vi "Display Results.vi"(8 "error in (no error)":errorcluster, 11 "Freq Sweet Result in":refnum<class "Freq Sweep Result.lvclass">) -> (0 "error out":errorcluster, 3 "Freq Sweet Result out":refnum<class "Freq Sweep Result.lvclass">)   [LabVIEW 2015, in "Frequency Measurement.lvlib" / "Freq Sweep Result.lvclass"]
uses:
  Freq Sweep Result.lvclass
  <userlib>/Common Components/Results/Results.lvclass
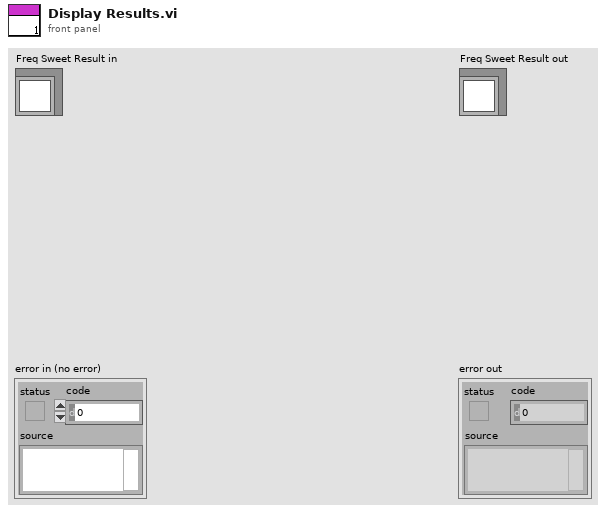
[diagram p1: front panel]
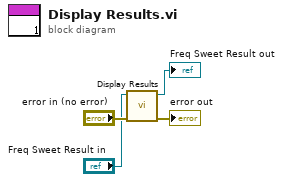
[diagram p0: block diagram]
diagram:
  n1 = call-parent "Display Results.vi"("error in (no error)"="error in (no error)", "Results in"="Freq Sweet Result in") -> ("error out"=→"error out":errorcluster, "Results out"=→"Freq Sweet Result out":refnum<class "Freq Sweep Result.lvclass">)  [unwired: 8 in]
